vi "P4CMD IsConnected to Provider.vi"(8 "error in (no error)":errorcluster) -> (0 "error out":errorcluster, 2 "active connection?":bool)   [LabVIEW 2020, in "NI_SCC_P4CMD.lvlib"]
uses:
  <vilib>/SourceControl/Providers/P4CMD/NI_SCC_P4CMD.lvlib
  <vilib>/SourceControl/Providers/P4CMD/P4CMD Mgr Functions.ctl
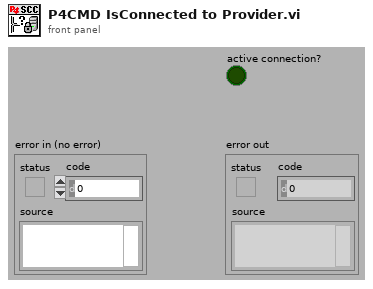
[diagram p1: front panel]
types:
  T1 = typedef "NI_SCC_P4CMD.lvlib/P4CMD Mgr Functions.ctl" = enum16{"Init", "Open", "Set Config Opts", "Initialized?", "IsRefValid?", "Get Config Opts", "Get Global Commands", "Close", "Uninit"}
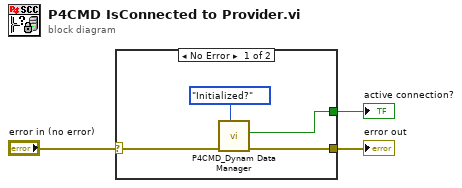
[diagram p0: block diagram]
diagram:
  n1 = case shown="No Error" "error in (no error)" {
    selector: "error in (no error)" -> [w6 w8]
    tunnel: [w5 w8] -> w2
    tunnel: [w4 _] -> w1
    frame No Error {
      n2 = call <vilib>:"P4CMD_Dynam Data Manager.vi"("function"=P4CMD_Mgr_Functions."Initialized?", "error in (no error)"=w6) -> ("error out"=w5:errorcluster, "initialized?"=w4:bool)  [unwired: 4 in, 4 out]
    }
    frame Error {
    }
  }
  "error out" <- w2
  "active connection?" <- w1
